vi "LatMan.vi"() -> ()   [LabVIEW 2014]
uses:
  <userlib>/Nanonis Prog Interface V5/Nanonis Prog Interface.lvlib
panel:
  out "Waveform Chart":sgl(graph)=-1.7974822e-08
  out "set":bool
  out "Time constant (s) old":sgl=0.00020079473 format="%#_6p"
  out "P-gain old":sgl=6.1516387e-12 format="%#_6p"
  out "I-gain old":sgl=3.0636453e-08 format="%#_6p"
  in  "Time constant (s)":sgl=0.001 caption="Time constant (s) (NaN = no change)" format="%#_6p"
  in  "P-gain":sgl=2e-12 caption="P-gain (NaN = no change)" format="%#_6p"
  in  "GO":bool
  in  "stop":bool
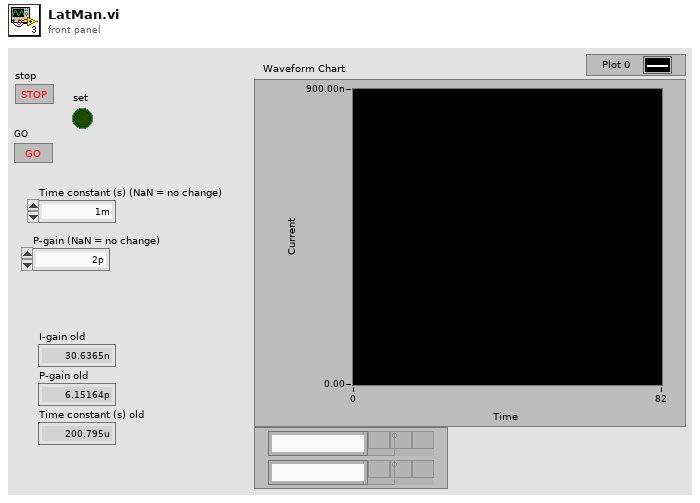
[diagram p1: front panel]
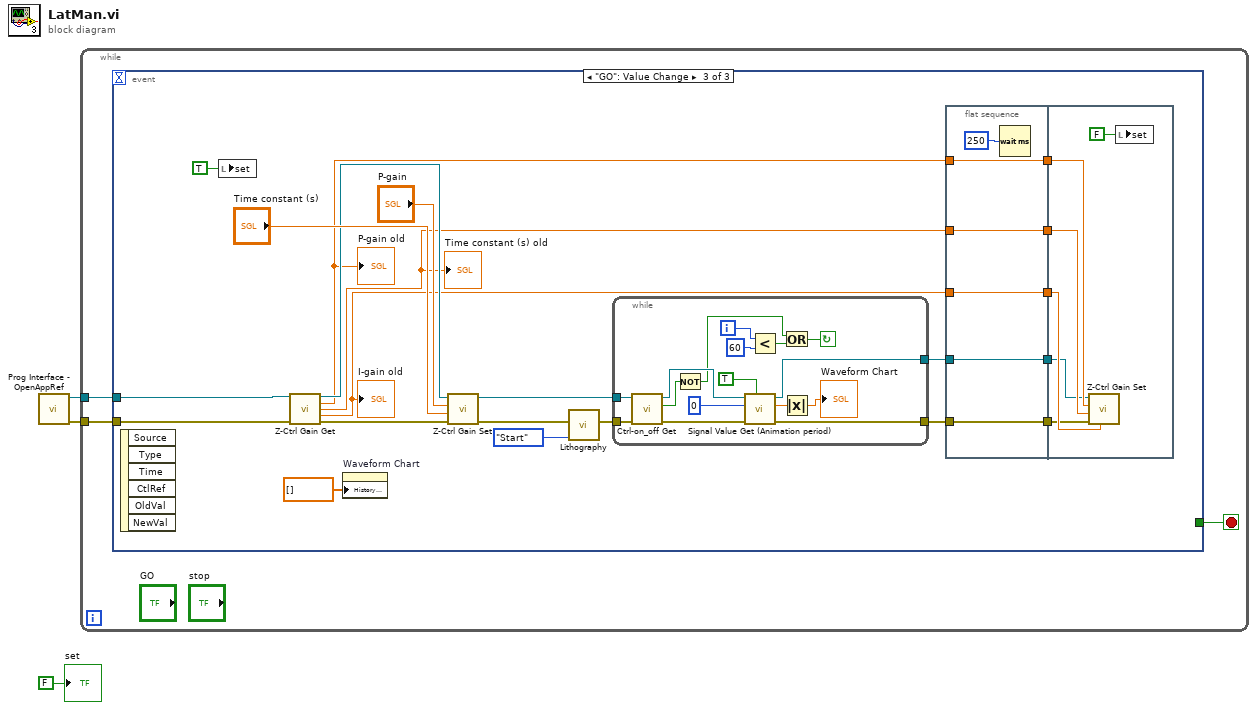
[diagram p0: block diagram]
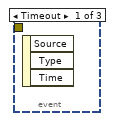
[diagram p2: hidden frame]
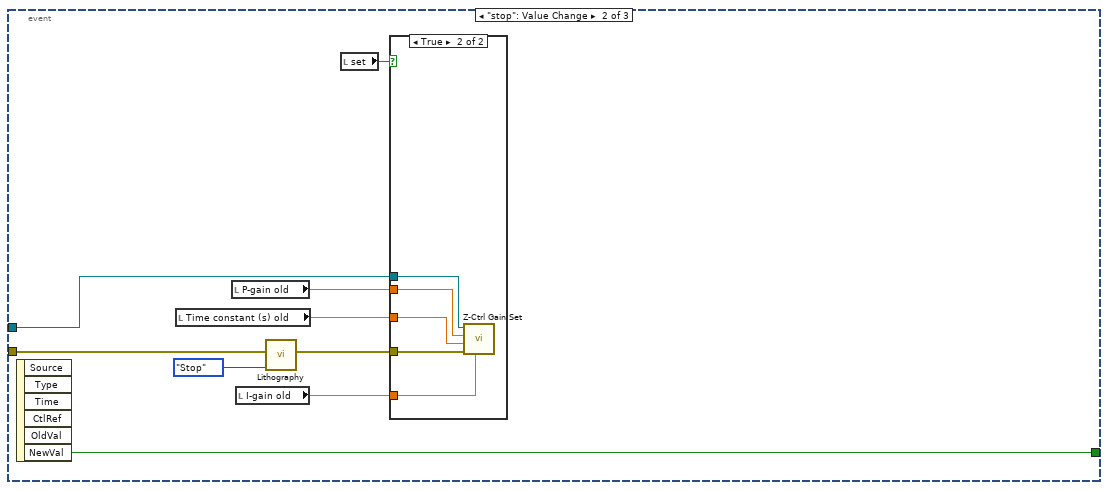
[diagram p3: hidden frame]
diagram:
  n1 = call <userlib>:"Prog Interface - OpenAppRef.vi"() -> ("Error out"=w2:errorcluster, "Application reference"=w3:refnum<vi>)  [unwired: 6 in]
  n2 = while {
    tunnel: w3 -> [w5]
    tunnel: w2 -> [w4]
    stop <- w6 stop-if-true
    n3 = event shown="[2] \"GO\": Value Change" {
      selector: _ -> [_ _ _]
      dyn-events: _ -> [_ _ _]
      timeout: _ -> [_ _ _]
      tunnel: [_ w15 _] -> w6
      tunnel: w5 -> [_ w12 w35]
      tunnel: w4 -> [_ w11 w36]
      event Timeout {
        n4 = event-data() -> ()  [unwired: 1 in, 3 out]
      }
      event "stop": Value Change {
        n5 = event-data() -> ("NewVal"=w15:bool)  [unwired: 1 in, 5 out]
        n6 = local read "Time constant (s) old"() -> (w9:sgl)
        n7 = local read "P-gain old"() -> (w8:sgl)
        n8 = local read "I-gain old"() -> (w10:sgl)
        n9 = call "Lithography.vi"("Enum"=enum16{"Stop", "Start"}."Stop", "error in (no error)"=w11) -> ("error out"=w13:errorcluster)  [unwired: 9 in]
        n10 = local read "set"() -> (w7:bool)
        n11 = case shown="True" w7 {
          tunnel: w13 -> [_ w20]
          tunnel: w12 -> [_ w19]
          tunnel: w10 -> [_ w18]
          tunnel: w9 -> [_ w17]
          tunnel: w8 -> [_ w16]
          frame False {
          }
          frame True {
            n12 = call <userlib>:"Z-Ctrl Gain Set.vi"("Integral"=w18, "error in (no error)"=w20, "Time constant (s)"=w17, "P-gain"=w16, "Application ref in"=w19) -> ()  [unwired: 4 in, 2 out]
          }
        }
      }
      event "GO": Value Change {
        n13 = event-data() -> ()  [unwired: 1 in, 6 out]
        n14 = local write "set"(TRUE ("set")) -> ()
        n15 = call <userlib>:"Z-Ctrl Gain Get.vi"("Application ref in"=w35, "error in (no error)"=w36) -> ("Application ref out"=w38:refnum<vi>, "P-gain"=w34:sgl, "Time constant (s)"=w33:sgl, "I-gain"=w32:sgl, "error out"=w37:errorcluster)  [unwired: 9 in]
        "I-gain old" <- w32
        "P-gain old" <- w34
        "Time constant (s) old" <- w33
        n16 = property on="Waveform Chart" class="WFChart (strict)"("History Data"=sgl[] []) -> ()  [unwired: 2 in, 2 out]
        n17 = call <userlib>:"Z-Ctrl Gain Set.vi"("error in (no error)"=w37, "Time constant (s)"="Time constant (s)", "P-gain"="P-gain", "Application ref in"=w38) -> ("error out"=w41:errorcluster, "Application ref out"=w28:refnum<vi>)  [unwired: 5 in]
        n18 = call "Lithography.vi"("Enum"=enum16{"Stop", "Start"}."Start", "error in (no error)"=w41) -> ("error out"=w30:errorcluster)  [unwired: 9 in]
        n19 = while {
          tunnel: w30 -> [w62]
          tunnel: [w67] -> w29
          tunnel: w28 -> [w64]
          tunnel: [w69] -> w27
          i -> [w57]
          stop <- w70 continue-if-true
          n20 = call <userlib>:"Ctrl-on_off Get.vi"("error in (no error)"=w62, "Application ref in"=w64) -> ("error out"=w61:errorcluster, "Z-Controller on/off status"=w59:bool, "Application ref out"=w63:refnum<vi>)  [unwired: 7 in]
          n21 = Not(x=w59) -> (.not. x?=w58:bool)
          n22 = call <userlib>:"Signal Value Get (Animation period).vi"("Wait for newest data (F=False)"=TRUE, "error in (no error)"=w61, "Signal index (0-47)"=i8 0, "Application ref in"=w63) -> ("error out"=w67:errorcluster, "Signal value"=w68:sgl, "Application ref out"=w69:refnum<vi>)  [unwired: 4 in]
          n23 = Less?(x=w57, y=60) -> (x < y?=w56:bool)
          n24 = Or(x=w58, y=w56) -> (x .or. y?=w70:bool)
          n25 = Absolute Value(x=w68) -> (abs(x)=→"Waveform Chart":sgl)
        }
        n26 = flat-sequence {
          tunnel: w27 -> [w44]
          tunnel: w29 -> [w45]
          tunnel: w32 -> [w46]
          tunnel: w33 -> [w47]
          tunnel: w34 -> [w48]
          tunnel: [w48] -> w26
          tunnel: [w47] -> w25
          tunnel: [w46] -> w24
          tunnel: [w45] -> w23
          tunnel: [w44] -> w22
          tunnel: w26 -> [w54]
          tunnel: w25 -> [w53]
          tunnel: w24 -> [w52]
          tunnel: w23 -> [w51]
          tunnel: w22 -> [w50]
          frame #0 {
            n27 = Wait (ms)(milliseconds to wait=u32 250) -> ()  [unwired: 1 out]
          }
          frame #1 {
            n28 = call <userlib>:"Z-Ctrl Gain Set.vi"("Integral"=w52, "error in (no error)"=w51, "Time constant (s)"=w53, "P-gain"=w54, "Application ref in"=w50) -> ()  [unwired: 4 in, 2 out]
            n29 = local write "set"(FALSE ("set")) -> ()
          }
        }
      }
    }
  }
  "set" <- FALSE ("set")
